vi "Handle Last Ack Core.vi"(4 "error in (no error)":errorcluster, 6 "Last Ack":refnum<class "Last Ack.lvclass">, 7 "Actor Nest in":refnum<class "Actor Nest.lvclass">) -> (0 "error out":errorcluster, 3 "Actor Nest out":refnum<class "Actor Nest.lvclass">)   [LabVIEW 2018, in "Actor Nest.lvlib" / "Actor Nest.lvclass"]
doc: "(<B>Filename</B>: Actor Framework.lvlib:Actor.lvclass:Handle Last Ack Core.vi)\n\nDefines how the caller actor responds to the Last Ack message from a nested actor. The Last Ack message is the final message a nested actor sends to its caller before it shuts down. The message contains information about the final state of the nested actor.\n\nBy default, this method does nothing except return any error the nested actor sent. A descendant class may override this method to define behavior."
uses:
  Actor Nest.lvclass
  <vilib>/ActorFramework/LastAck/Last Ack.lvclass
  <vilib>/ActorFramework/LastAck/Last Ack.lvclass/Last Ack.ctl
  Actor Nest.lvclass/Actor Nest.ctl
  <vilib>/ActorFramework/Actor/Actor.lvclass
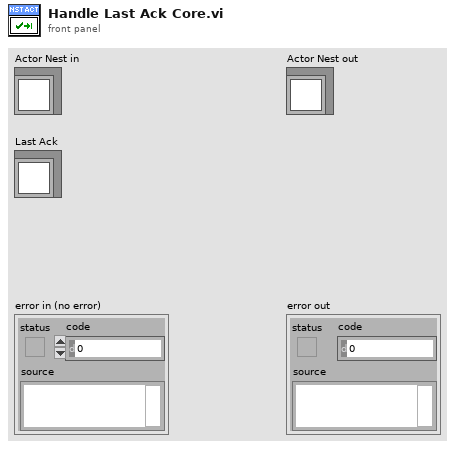
[diagram p1: front panel]
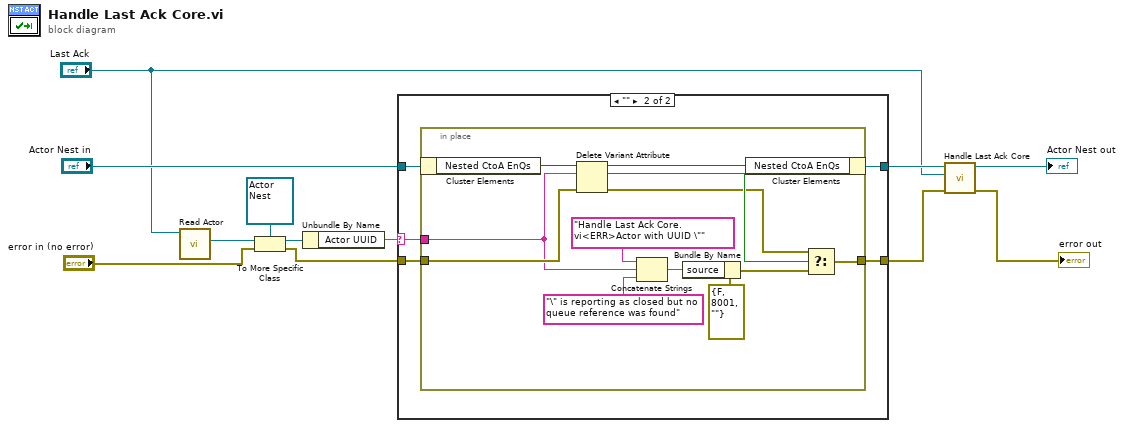
[diagram p0: block diagram]
diagram:
  n1 = call <vilib>:"Read Actor.vi"("Last Ack"="Last Ack") -> ("Actor"=w5:refnum<class "Actor.lvclass">)  [unwired: 10 in]
  n2 = To More Specific Class(target class=refnum<class "Actor Nest.lvclass"> refnum ("Actor Nest.lvlib:Actor Nest.lvclass"), reference=w5, error in="error in (no error)") -> (specific class reference=w4:refnum<class "Actor Nest.lvclass">, error out=w2:errorcluster)
  n3 = Unbundle By Name(w4) -> ("Actor UUID"=w1:string)
  n4 = case shown="\"\"" w1 {
    selector: w1 -> [_ w15]
    tunnel: [w14 w19] -> w12
    tunnel: "Actor Nest in" -> [w14 w18]
    tunnel: [w13 w17] -> w9
    tunnel: w2 -> [w13 w16]
    frame Default {
    }
    frame "" {
      n5 = in-place {
        in-place-border: w16 -> [w31]
        in-place-border: [w21] -> w17
        in-place-border: w15 -> [w20]
        n6 = in-place-cluster #1(w18) -> ("Nested CtoA EnQs"=w30:variant)
        n7 = Delete Variant Attribute(4:w31, 6:w20, 7:w30) -> (0:w23:errorcluster, 2:w24:bool, 3:w29:variant)
        n8 = Concatenate Strings("Handle Last Ack Core.vi<ERR>Actor with UUID \"" ("source"), w20, "\" is reporting as closed but no queue reference was found") -> (w27:string)
        n9 = Bundle By Name(cluster=errorcluster {"status"=FALSE, "code"=8001, "source"=""} ("error out"), "source"=w27) -> (w22:errorcluster)
        n10 = in-place-cluster #1("Nested CtoA EnQs"=w29) -> (w19:refnum<class "Actor Nest.lvclass">)
        n11 = Select(t=w23, s=w24, f=w22) -> (s? t:f=w21:errorcluster)
      }
    }
  }
  n12 = call-parent "Handle Last Ack Core.vi"("error in (no error)"=w9, "Last Ack"="Last Ack", "Actor in"=w12) -> ("error out"=→"error out":errorcluster, "Actor out"=→"Actor Nest out":refnum<class "Actor Nest.lvclass">)  [unwired: 3 in]
